vi "Calculate Trigger Settings.vi"(0 "trigger source":u8, 1 "actual channel configuration":T1[](array[typedef]) {"vertical offset" format="%_3p"; "vertical range" format="%_3p"}, 5 "trigger slope":T5, 7 "level (V)":dbl, 9 "hysteresis (%fs)":dbl=0.25, 11 "error in":errorcluster) -> (4 "high level (V)":dbl, 6 "low level (V)":dbl, 15 "error out":errorcluster)   [LabVIEW 2021, in "Device Session.lvclass"]
uses:
  Device Session.lvclass
  <instrlib>/_niInstr/Data Trigger/v1/Shared/Public/Edge Configuration Trigger Slope.ctl
  <instrlib>/HSAI-RIO/Types/v1/Host/Typedefs/Channel Configuration.ctl
  <instrlib>/HSAI-RIO/Types/v1/Host/Typedefs/Coupling.ctl
  <instrlib>/HSAI-RIO/Types/v1/Host/Typedefs/Impedance.ctl
  <instrlib>/HSAI-RIO/Types/v1/Host/Typedefs/Bandwidth.ctl
  <vilib>/Utility/error.llb/Error Cluster From Error Code.vi
  <vilib>/ErrorRing/Error Ring.xnode
  <instrlib>/_niInstr/Data Trigger/v1/Shared/niInstr Data Trigger v1 Shared.lvlib
  <instrlib>/HSAI-RIO/Types/v1/Host/niHSAI Types v1 Host.lvlib
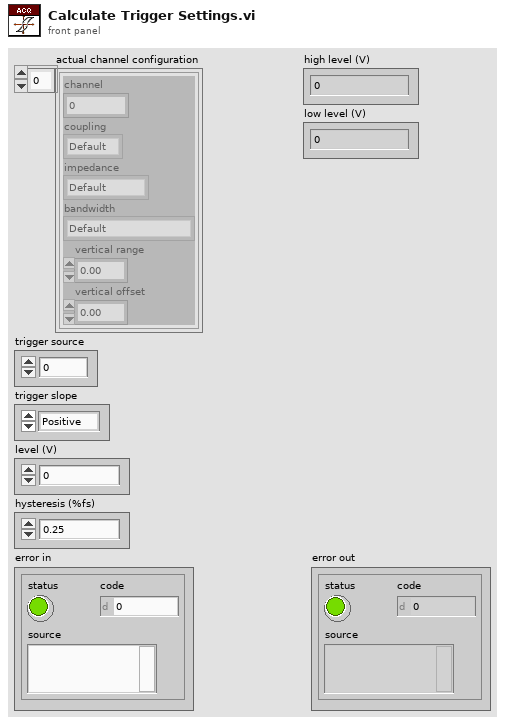
[diagram p1: front panel]
types:
  T1 = typedef "niHSAI Types v1 Host.lvlib/Channel Configuration.ctl" = cluster{"channel":u32, "coupling":T2, "impedance":T3, "bandwidth":T4, "vertical range":dbl, "vertical offset":dbl}
  T2 = typedef "niHSAI Types v1 Host.lvlib/Coupling.ctl" = enum8{"Default", "DC", "AC"}
  T3 = typedef "niHSAI Types v1 Host.lvlib/Impedance.ctl" = enum8{"Default", "1 mega ohm", "50 ohm"}
  T4 = typedef "niHSAI Types v1 Host.lvlib/Bandwidth.ctl" = enum8{"Default", "Full Bandwidth", "Anti-alias Filter", "150 MHz"}
  T5 = typedef "niInstr Data Trigger v1 Shared.lvlib/Edge Configuration Trigger Slope.ctl" = enum8{"Positive", "Negative"}
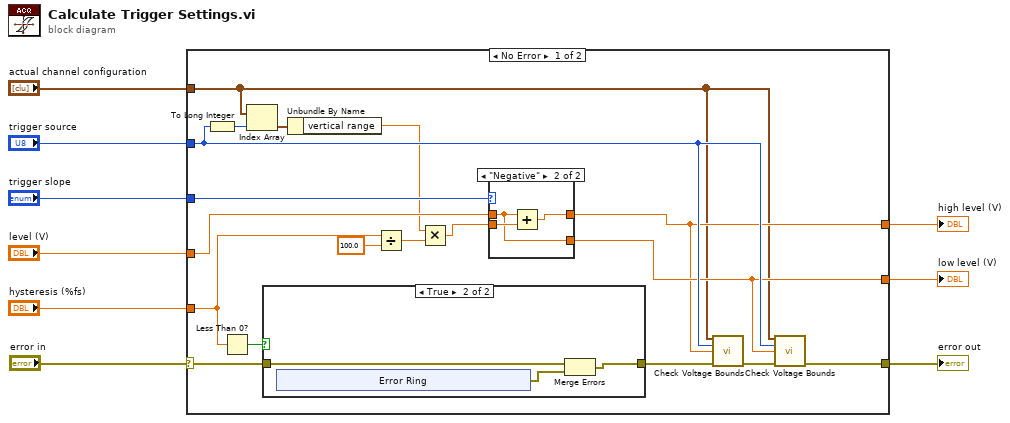
[diagram p0: block diagram]
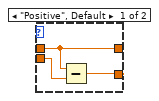
[diagram p3: hidden frame]
diagram:
  n1 = case shown="No Error" "error in" {
    selector: "error in" -> [w23 w42]
    tunnel: "actual channel configuration" -> [w10 _]
    tunnel: "trigger source" -> [w20 _]
    tunnel: "trigger slope" -> [w27 _]
    tunnel: "level (V)" -> [w26 _]
    tunnel: "hysteresis (%fs)" -> [w17 _]
    tunnel: [w21 w42] -> w3
    tunnel: [w11 _] -> w2
    tunnel: [w12 _] -> w1
    frame No Error {
      n2 = To Long Integer(number=w20) -> (32bit integer=w19:i32)
      n3 = Less Than 0?(x=w17) -> (x < 0?=w25:bool)
      n4 = Index Array(array=w10, index=w19) -> (element=w18:T1)
      n5 = case shown="True" w25 {
        tunnel: [w28 w29] -> w24
        tunnel: w23 -> [w28 w31]
        frame False {
        }
        frame True {
          n6 = xnode "Error Ring"() -> ("error out"=w30:errorcluster)
          n7 = Merge Errors(w31, w30) -> (w29:errorcluster)
        }
      }
      n8 = Unbundle By Name(w18) -> ("vertical range"=w14:dbl)
      n9 = Divide(x=w17, y=100.0) -> (x/y=w15:dbl)
      n10 = Multiply(x=w14, y=w15) -> (x*y=w13:dbl)
      n11 = case shown="\"Negative\"" w27 {
        tunnel: w13 -> [w38 w41]
        tunnel: w26 -> [w37 w39]
        tunnel: [w37 w40] -> w11
        tunnel: [w36 w39] -> w12
        frame "Positive", Default {
          n12 = Subtract(x=w37, y=w38) -> (x-y=w36:dbl)
        }
        frame "Negative" {
          n13 = Add(x=w39, y=w41) -> (x+y=w40:dbl)
        }
      }
      n14 = call "Check Voltage Bounds.vi"("channel configuration"=w10, "trigger source"=w20, "level (V)"=w11, "error in"=w24) -> ("error out"=w22:errorcluster)  [unwired: 11 in]
      n15 = call "Check Voltage Bounds.vi"("channel configuration"=w10, "trigger source"=w20, "level (V)"=w12, "error in"=w22) -> ("error out"=w21:errorcluster)  [unwired: 11 in]
    }
    frame Error {
    }
  }
  "error out" <- w3
  "high level (V)" <- w2
  "low level (V)" <- w1
